vi "SaveHands.vi"(8 "error in (no error)":errorcluster, 11 "Controller Refnum":refnum<k24>) -> (0 "error out":errorcluster, 3 "Hand array":T1[](array[typedef]))   [LabVIEW 2017, in "LeapMotion.lvlib"]
uses:
  TypeDefs/LEAPhand.ctl
  TypeDefs/LEAPvector.ctl
  TypeDefs/LEAPfinger.ctl
  TypeDefs/LEAPbone.ctl
  C:/Users/snordinh/Desktop/LEAP/LEAP-sign-language-test/LeapMotion/Dynamic Libraries/LeapCSharp.NET4.5.dll
  Dynamic Libraries/LeapCSharp.NET4.5.dll
  LeapMotion.lvlib
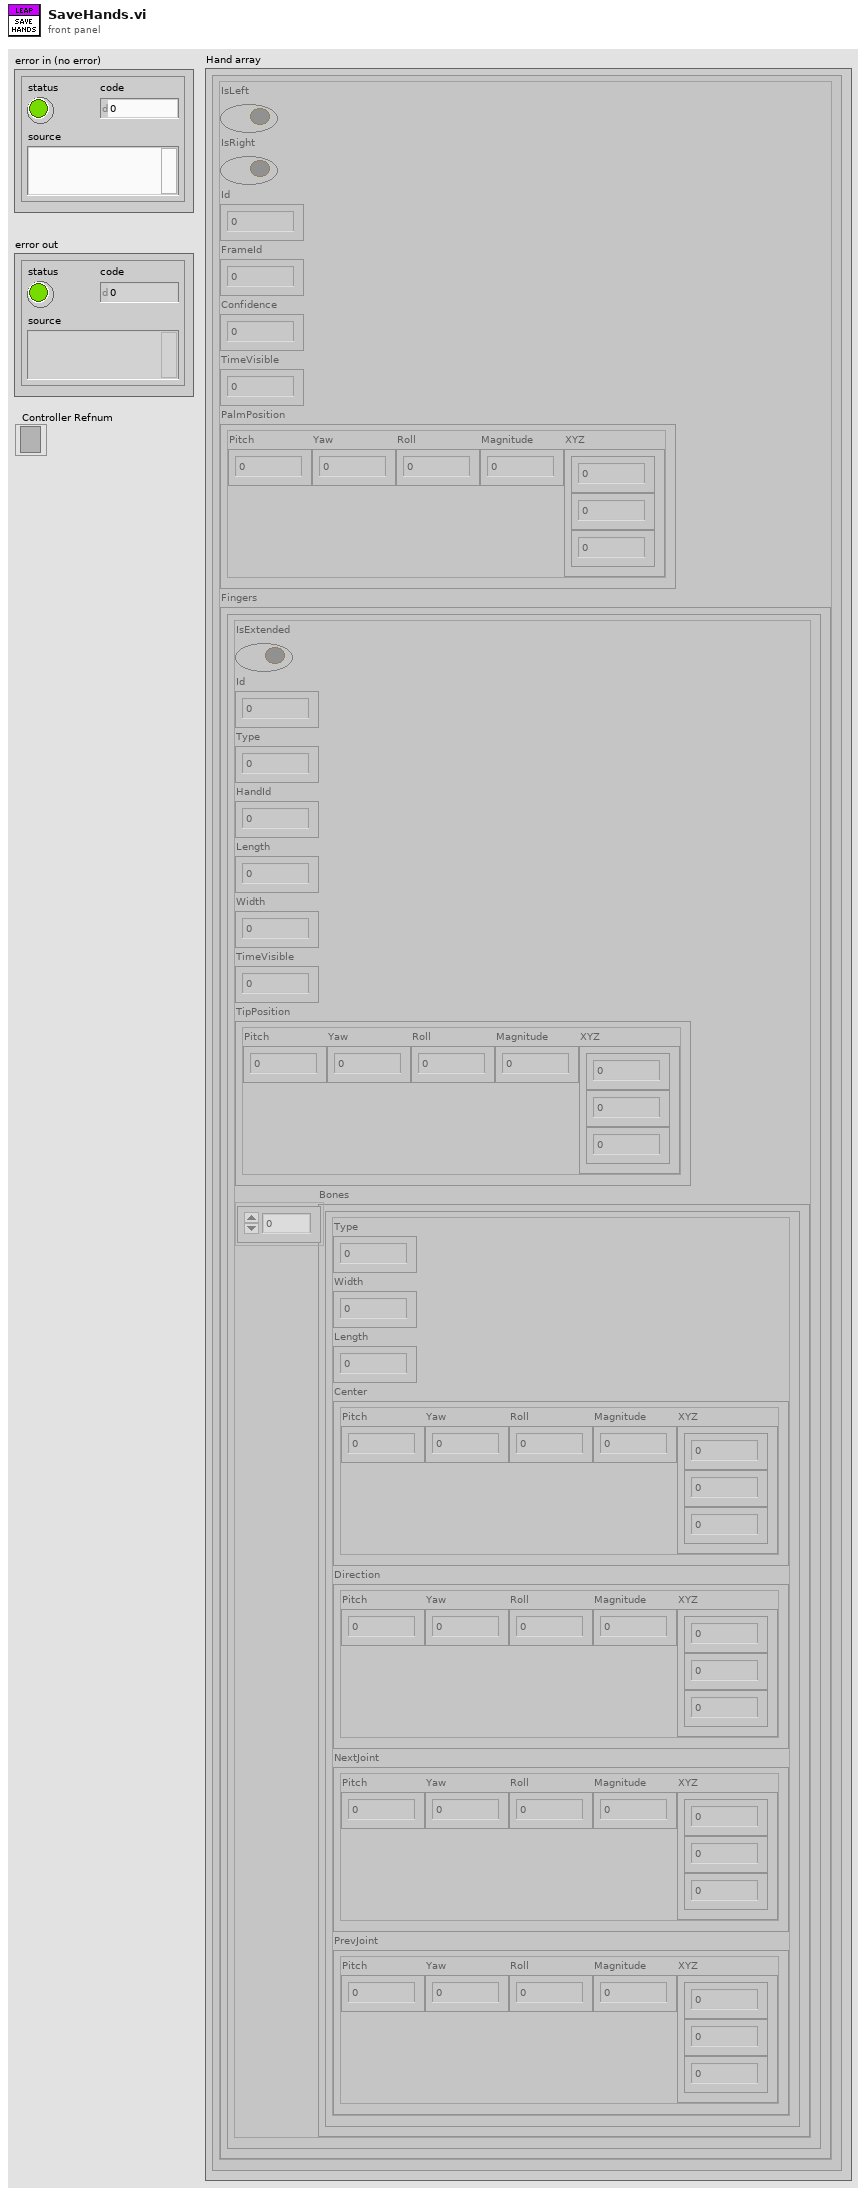
[diagram p1: front panel]
types:
  T1 = typedef "LeapMotion.lvlib/LEAPhand.ctl" = cluster{"IsLeft":bool, "IsRight":bool, "Id":i32, "FrameId":i64, "Confidence":sgl, "TimeVisible":sgl, "PalmPosition":T2, "Fingers":T3[]}
  T2 = typedef "LeapMotion.lvlib/LEAPvector.ctl" = cluster{"Pitch":sgl, "Yaw":sgl, "Roll":sgl, "Magnitude":sgl, "XYZ":sgl[]}
  T3 = typedef "LeapMotion.lvlib/LEAPfinger.ctl" = cluster{"IsExtended":bool, "Id":i32, "Type":i32, "HandId":i32, "Length":sgl, "Width":sgl, "TimeVisible":sgl, "TipPosition":T2, "Bones":T4[]}
  T4 = typedef "LeapMotion.lvlib/LEAPbone.ctl" = cluster{"Type":i32, "Width":sgl, "Length":sgl, "Center":T2, "Direction":T2, "NextJoint":T2, "PrevJoint":T2}
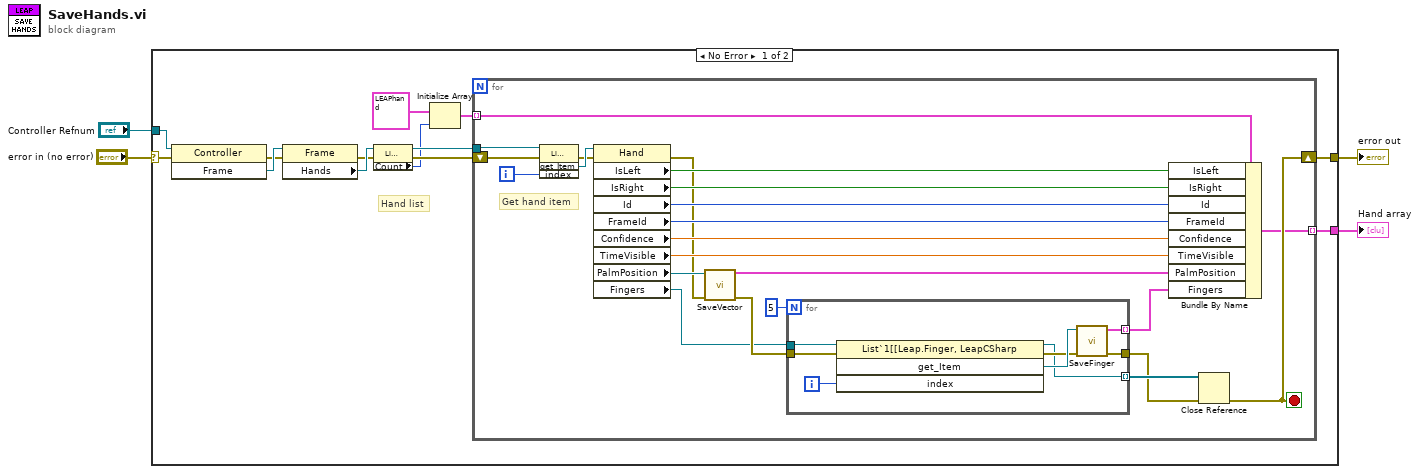
[diagram p0: block diagram]
diagram:
  n1 = case shown="No Error" "error in (no error)" {
    selector: "error in (no error)" -> [w7 w49]
    tunnel: [w15 w49] -> w2
    tunnel: [w11 _] -> w4
    tunnel: "Controller Refnum" -> [w9 _]
    frame No Error {
      # "Hand list"
      n2 = invoke class="Controller" method="Frame"(reference=w9, error in=w7) -> (error out=w6:errorcluster, "Frame"=w10:refnum<k24>)  [unwired: 1 in, 1 out]
      n3 = property class="Frame"(reference=w10, error in=w6) -> (error out=w5:errorcluster, "Hands"=w8:refnum<k24>)  [unwired: 1 out]
      n4 = property class="List`1[[Leap.Hand, LeapCSharp.N"(reference=w8, error in=w5) -> (reference out=w17:refnum<k24>, error out=w16:errorcluster, "Count"=w14:i32)
      n5 = Initialize Array(T1 {"IsLeft"=FALSE, "IsRight"=FALSE, "Id"=0, "FrameId"=0, "Confidence"=0.0, "TimeVisible"=0.0, "PalmPosition"={"Pitch"=0.0, "Yaw"=0.0, "Roll"=0.0, "Magnitude"=0.0, "XYZ"=[]}, "Fingers"=[]} ("Hand"), w14) -> (w12:T1[])
      n6 = for {
        tunnel: w17 -> [w40]
        tunnel: w12 -> [w24] mode=indexing
        tunnel: [w19] -> w11 mode=indexing
        shift-right: [w21] -> w15
        shift-left: w16 -> [w39]
        i -> [w20]
        stop <- w21 stop-if-true
        # "Get hand item"
        n7 = invoke class="List`1[[Leap.Hand, LeapCSharp.N" method="get_Item"(reference=w40, error in=w39, "index"=w20) -> (error out=w37:errorcluster, "get_Item"=w38:refnum<k24>)  [unwired: 1 in, 2 out]
        n8 = property class="Hand"(reference=w38, error in=w37) -> (error out=w28:errorcluster, "IsLeft"=w35:bool, "IsRight"=w34:bool, "Id"=w33:i32, "FrameId"=w32:i64, "Confidence"=w31:sgl, "TimeVisible"=w30:sgl, "PalmPosition"=w36:refnum<k24>, "Fingers"=w18:refnum<k24>)  [unwired: 1 out]
        n9 = call "SaveVector.vi"("error in (no error)"=w28, "Vector Refnum"=w36) -> ("error out"=w25:errorcluster, "LEAPvector"=w29:T2)  [unwired: 8 in]
        n10 = for {
          N: 5 -> [_]
          tunnel: [w48] -> w22
          tunnel: w18 -> [w45]
          tunnel: [w44] -> w26 mode=indexing
          tunnel: w25 -> [w42]
          tunnel: [w41] -> w23 mode=indexing
          i -> [w43]
          n11 = invoke class="List`1[[Leap.Finger, LeapCSharp" method="get_Item"(reference=w45, error in=w42, "index"=w43) -> (reference out=w41:refnum<k24>, error out=w46:errorcluster, "get_Item"=w47:refnum<k24>)  [unwired: 1 in, 1 out]
          n12 = call "SaveFinger.vi"("error in (no error)"=w46, "Finger Refnum"=w47) -> ("error out"=w48:errorcluster, "Finger"=w44:T3)  [unwired: 8 in]
        }
        n13 = Bundle By Name(cluster=w24, "IsLeft"=w35, "IsRight"=w34, "Id"=w33, "FrameId"=w32, "Confidence"=w31, "TimeVisible"=w30, "PalmPosition"=w29, "Fingers"=w26) -> (w19:T1)
        n14 = Close Reference(reference=w23, error in (no error)=w22) -> (error out=w21:errorcluster)
      }
    }
    frame Error {
    }
  }
  "Hand array" <- w4
  "error out" <- w2
